vi "Data_get.vi"() -> ()   [LabVIEW 2009]
uses:
  <vilib>/Analysis/2dsp.llb/Real FFT.vi
  <vilib>/Analysis/NI_AALPro.lvlib
panel:
  in  "autoOFF":bool caption="Auto switch OFF"
  in  "SetRP":bool
  in  "Rep.Period":dbl=1.0 caption="Repetition Period(c)" min=1e-06 max=1000.0 step=0.1
  in  "PauseB":bool caption="Pause"
  in  "Substr":bool
  out "tdsavges#":i32 caption="tds averaged:"
  in  "Auto":bool caption="Autosave"
  in  "FFT every#":u32=1 min=1 max=1000 step=1
  in  "#steps":u32=1 min=1 step=1
  in  "f step (MHz)":dbl=0.0003 min=0.00025 max=67.0 step=1e-06 format="%#.12f"
  in  "ps/point":T1(ring)
  in  "ns/div":T2(ring)
  out "Current sweep":u32=1 min=1 max=1000 step=1
  in  "Ext":string="ccd"
  out "f cur. (MHz)":string
  in  "Name":string="trace"
  in  "Folder":path
  in  "#Sweeps":u32=1 min=1 max=1000 step=1
  in  "Ampl. (dBm)":dbl min=-135.0 max=30.0 step=0.5 format="%#_8g"
  in  "f start (MHz)":dbl=0.0003 min=0.00025 max=67.0 step=1e-06 format="%#.12f"
  in  "Start":bool
  in  "Quit":bool
  in  "E8257D VISA Port":refnum<visa-resource-name>="GPIB0::1::INSTR"
  out "read time (ms)":u32
  out "#points":u32
  out "Busy":bool
  in  "Repetition rate (Hz)":ext=2.5
  in  "Chirp start (MHz)":ext=2.5
  in  "Filter up to (MHz)":ext=2.5
  in  "Amount of averagings":u32=10 min=1 step=1
  out "Data":dbl[](array[numeric])
  out "XY Graph 5":cluster{ext[], dbl[]}(graph)
  out "FFT (Im)":dbl[](array[numeric])
  out "FFT (Re)":dbl[](array[numeric])
  out "Final array":ext[][](array[numeric])
  out "size(s)":i32
  out "Oscilloscope Data":dbl[](array[numeric])
  in  "Channel Number":u16=1
  out "Oscilloscope graph":dbl[](graph)
  in  "Stop":bool
  in  "TDS VISA Port":refnum<visa-resource-name>="GPIB0::1::INSTR"
  # "TDS6000"
  # "DG645"
  # "E8257D"
  # "File Storage"
  # "Control"
  # "Spectrum data"
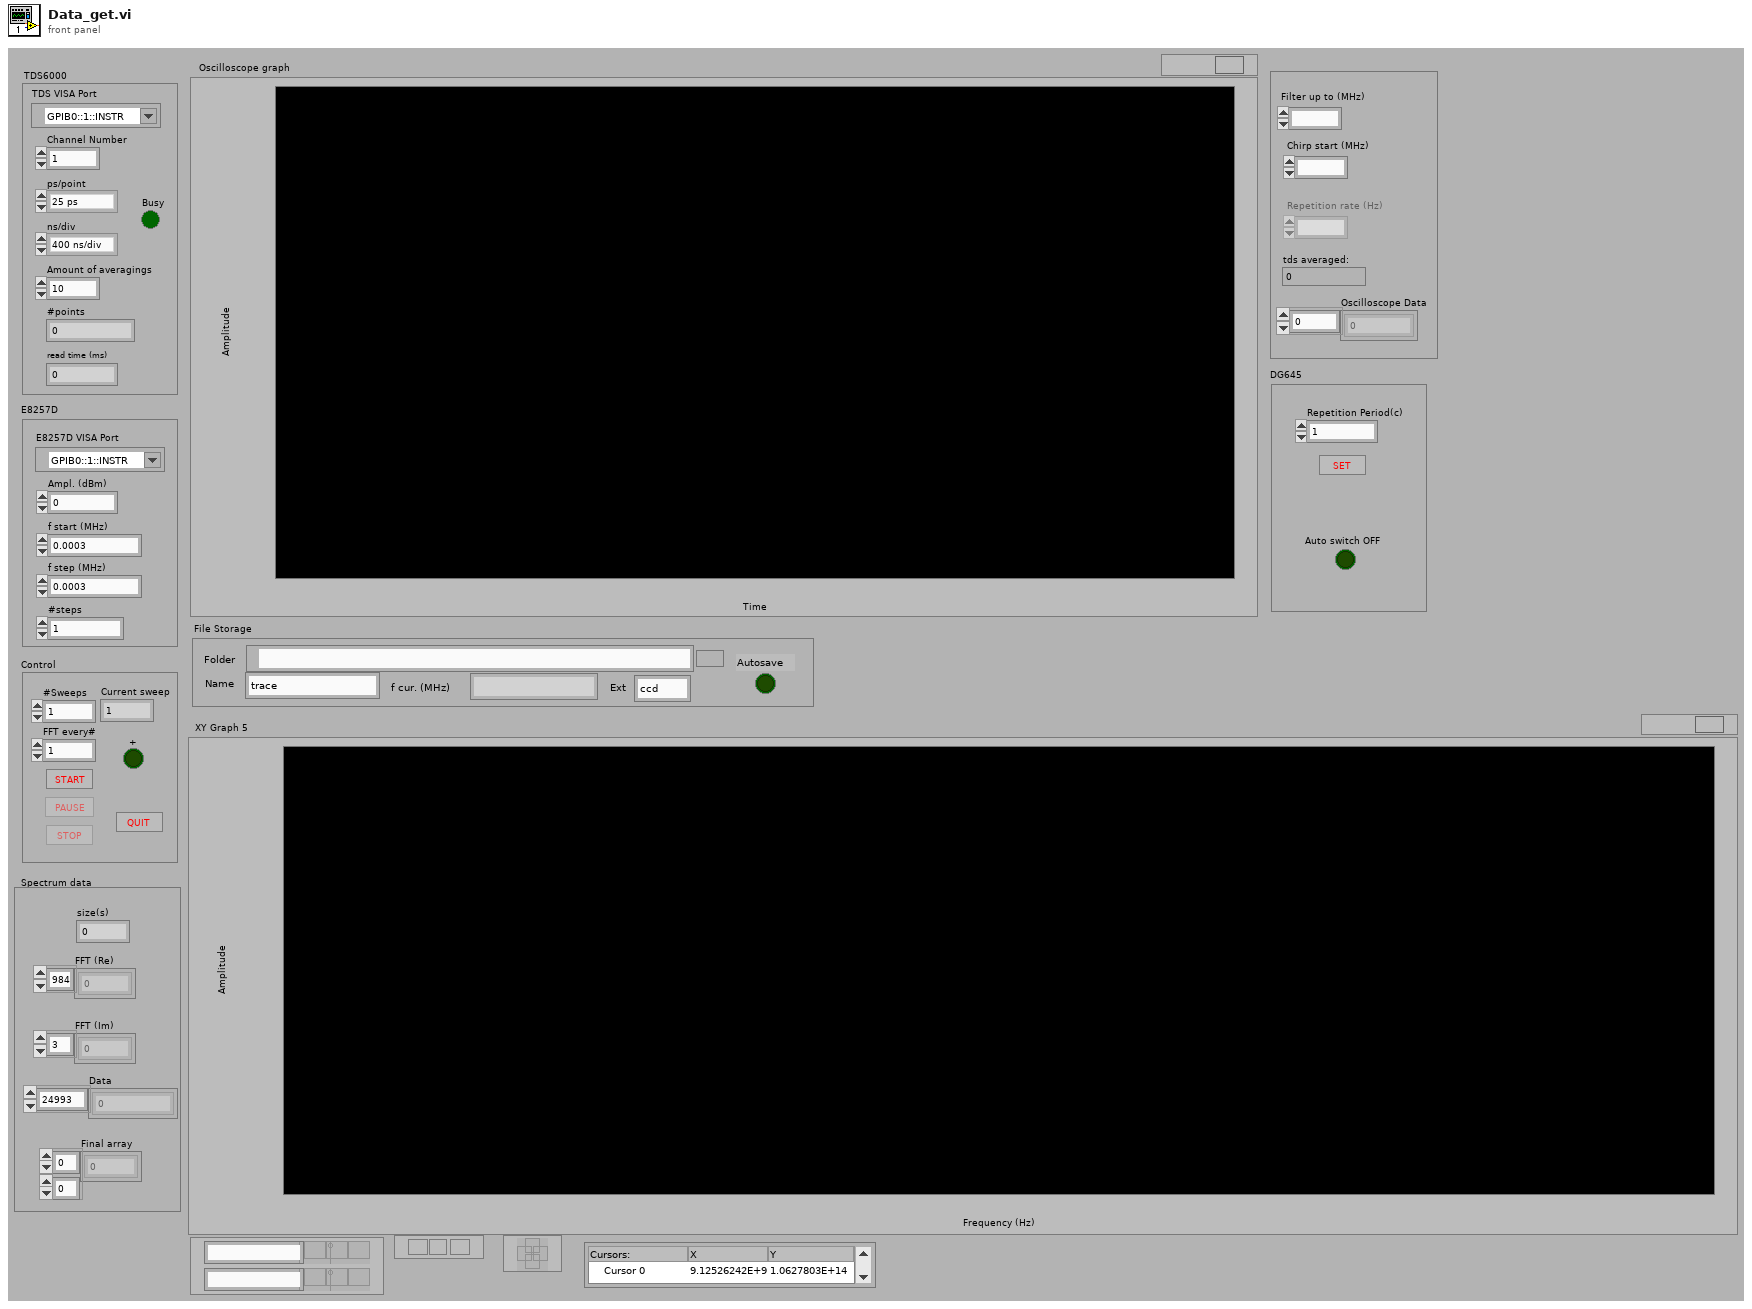
[diagram p1: front panel]
types:
  T1 = enum16{"25 ps", "50 ps", "100 ps", "200 ps", "400 ps", "800 ps", "2 ns"}
  T2 = enum16{"400 ns/div", "1 us/div", "2 us/div", "4 us/div", "10 us/div", "20 us/div"}
  T3 = enum8{"Enabled", "Disabled", "Disabled and Grayed Out"}
  T4 = enum16{"open", "replace", "create", "open or create", "replace or create", "replace or create with confirmation"}
  T5 = cluster{"Folder":path, "Name":string, "Ext":string}
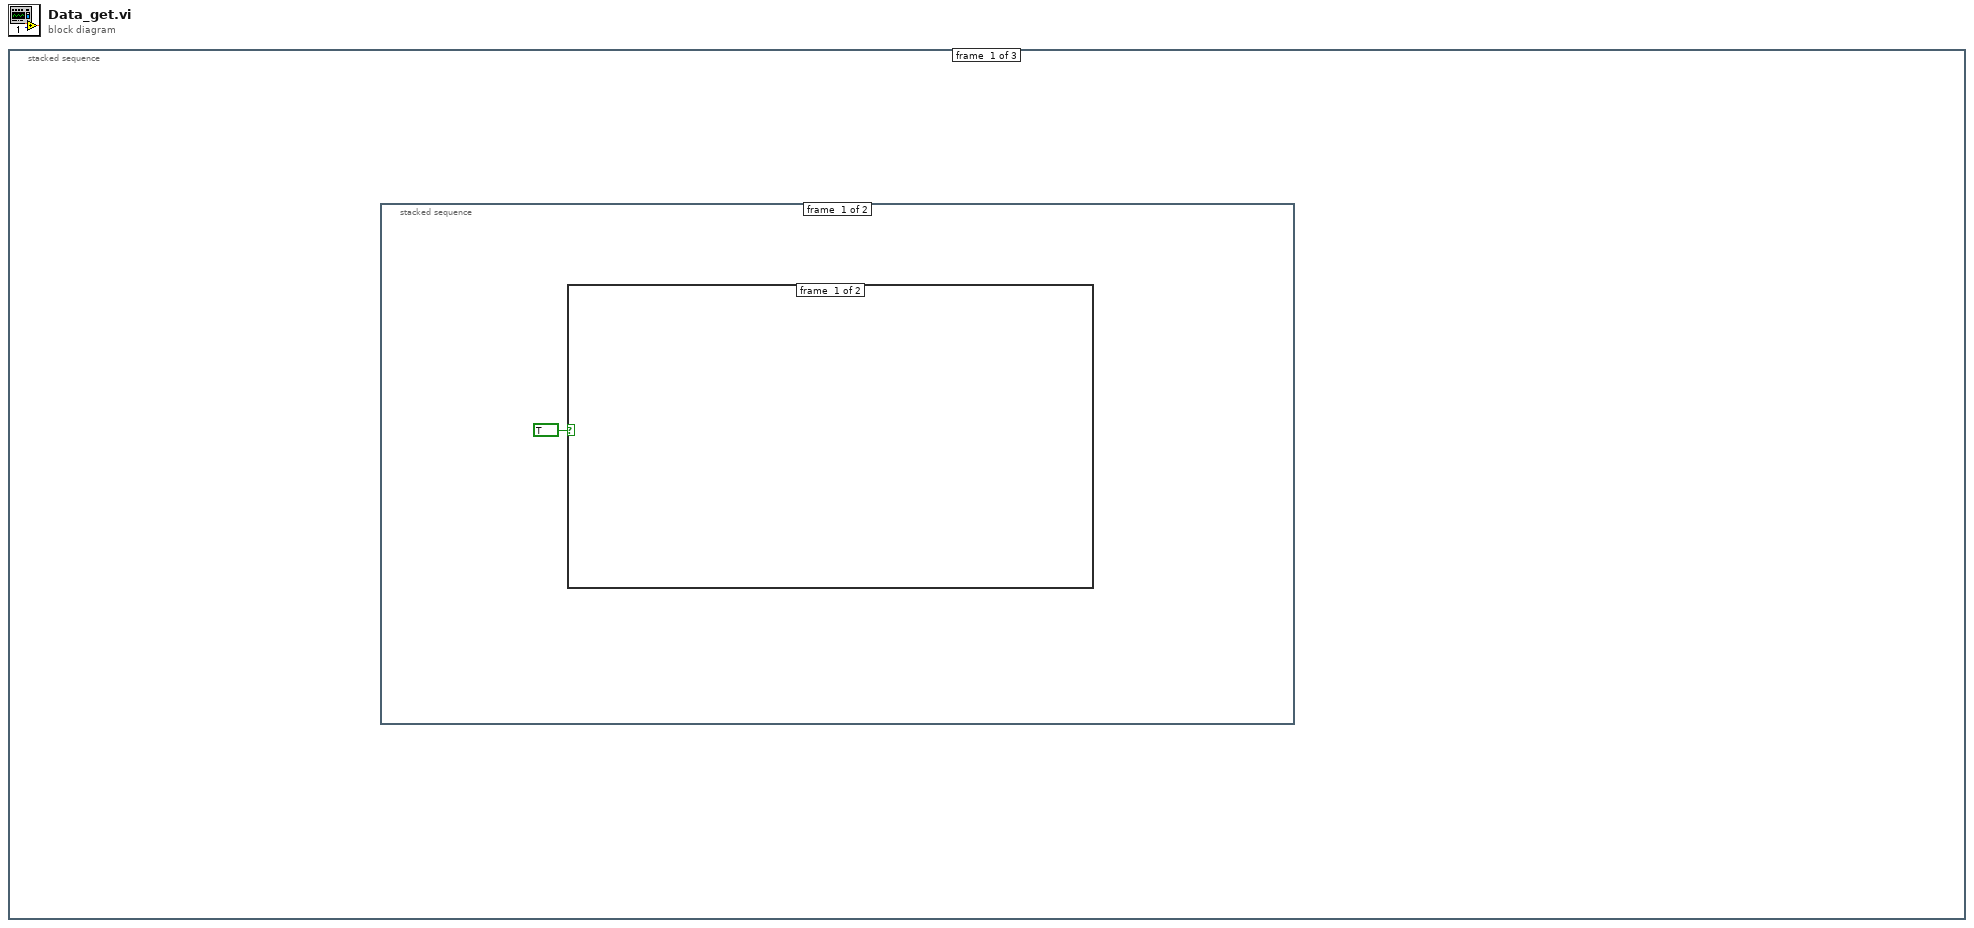
[diagram p0: block diagram]
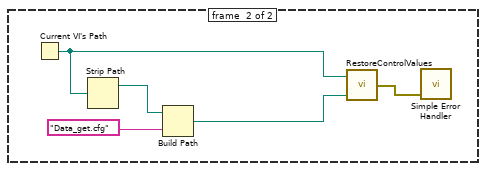
[diagram p2: hidden frame]
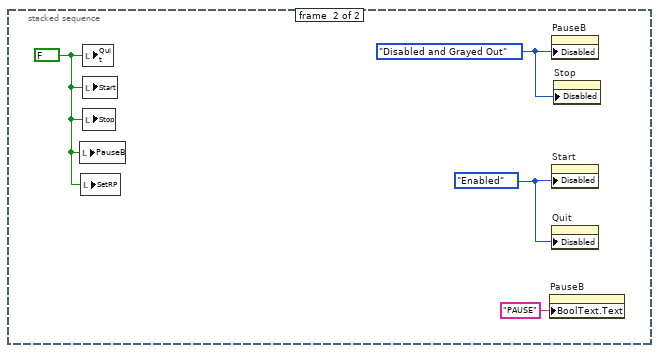
[diagram p3: hidden frame]
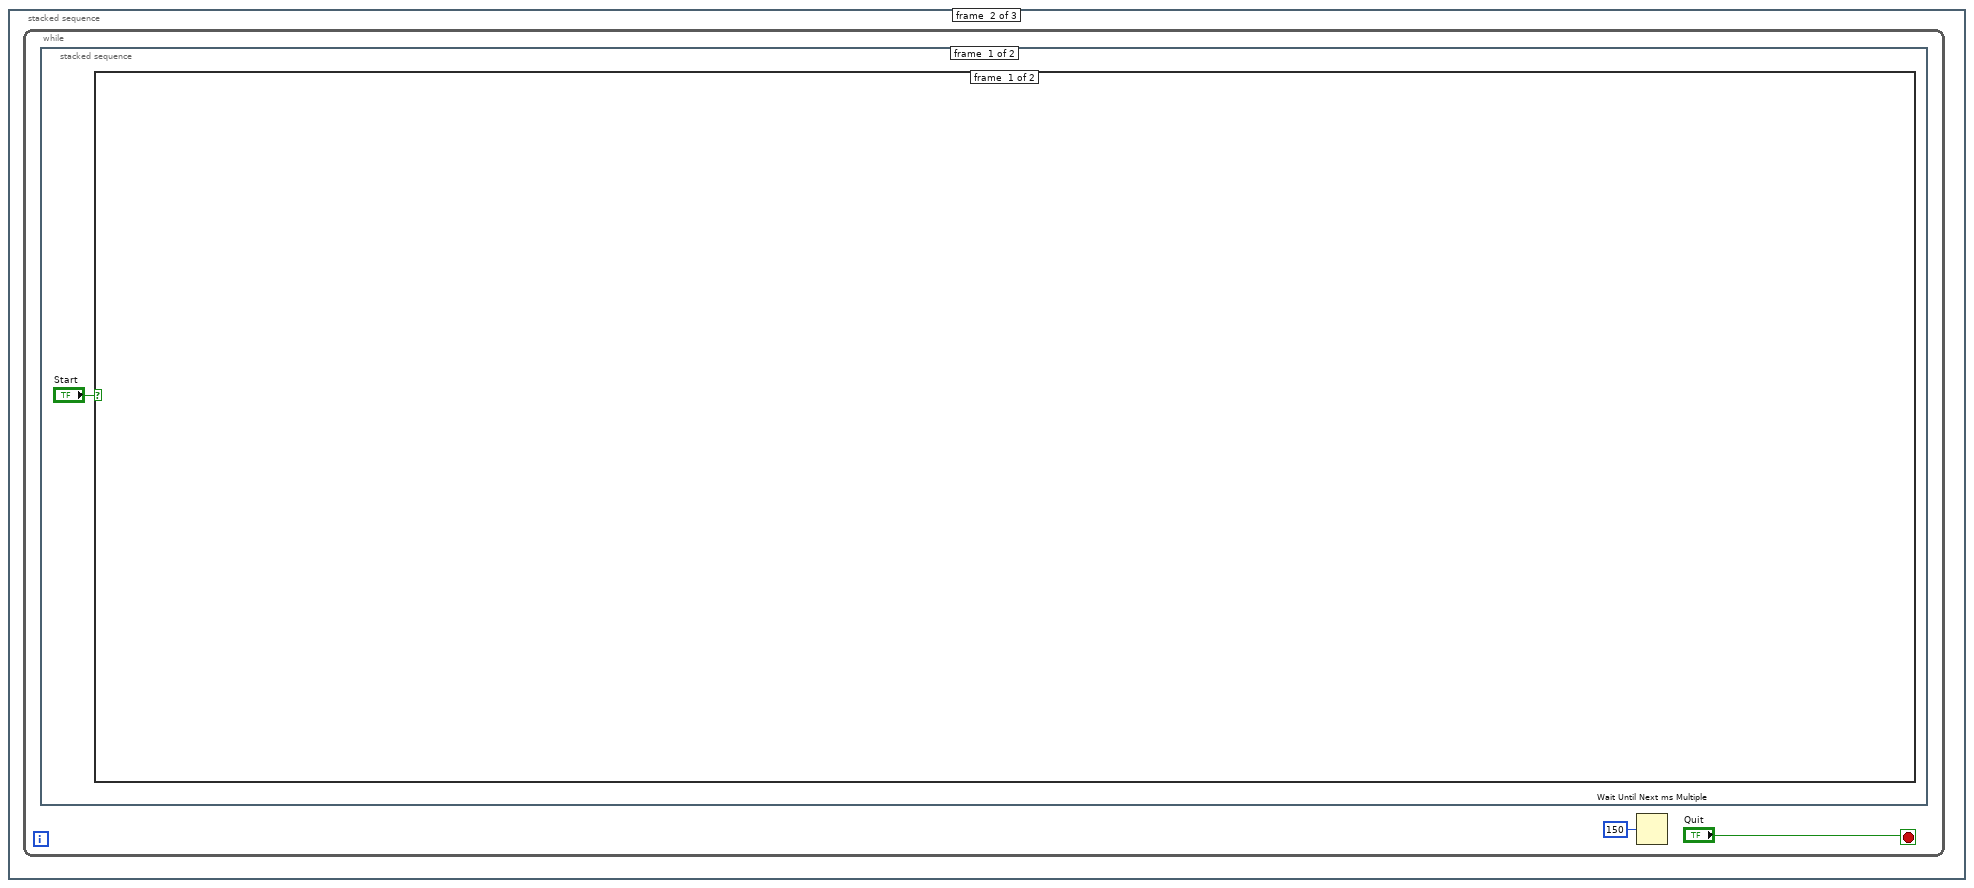
[diagram p4: hidden frame]
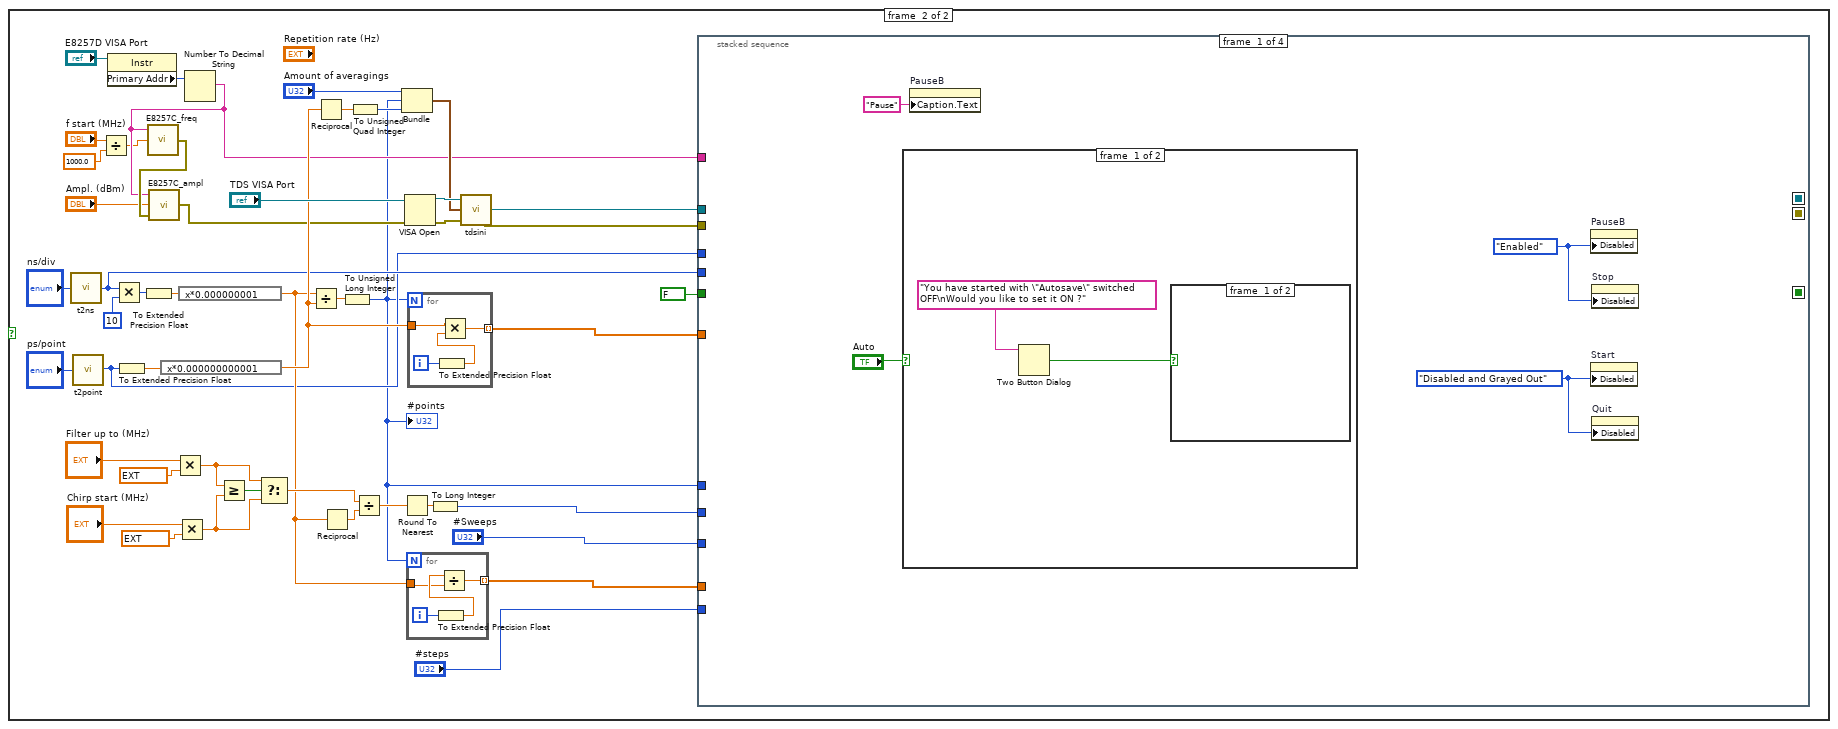
[diagram p5: hidden frame]
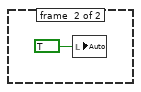
[diagram p6: hidden frame]
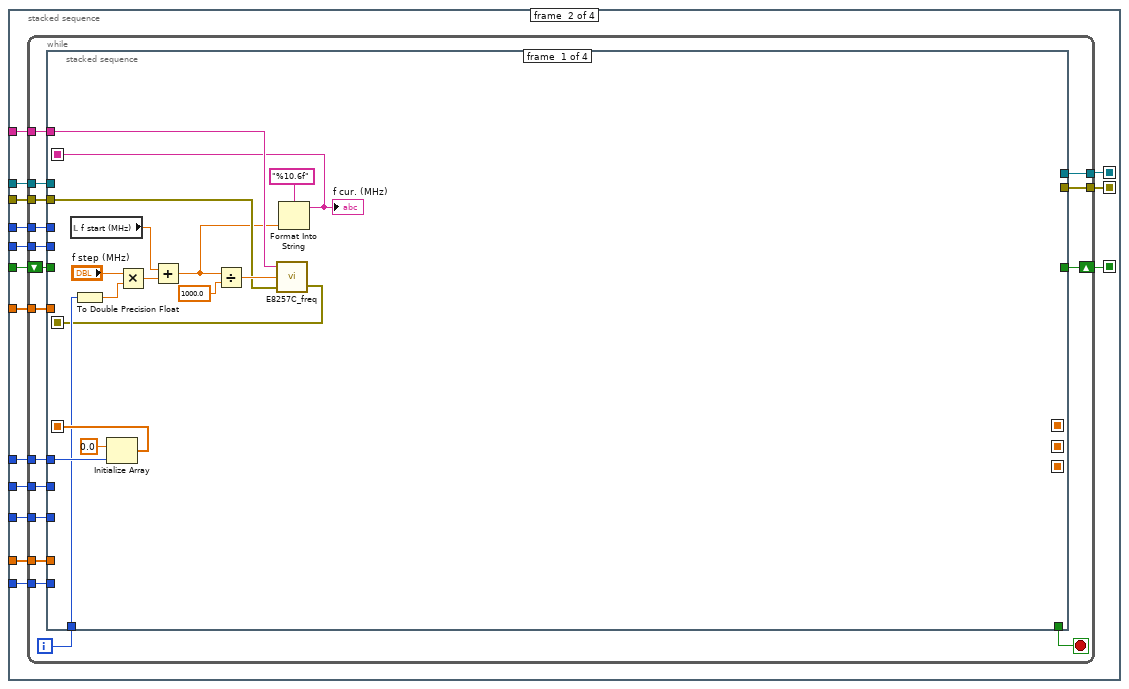
[diagram p8: hidden frame]
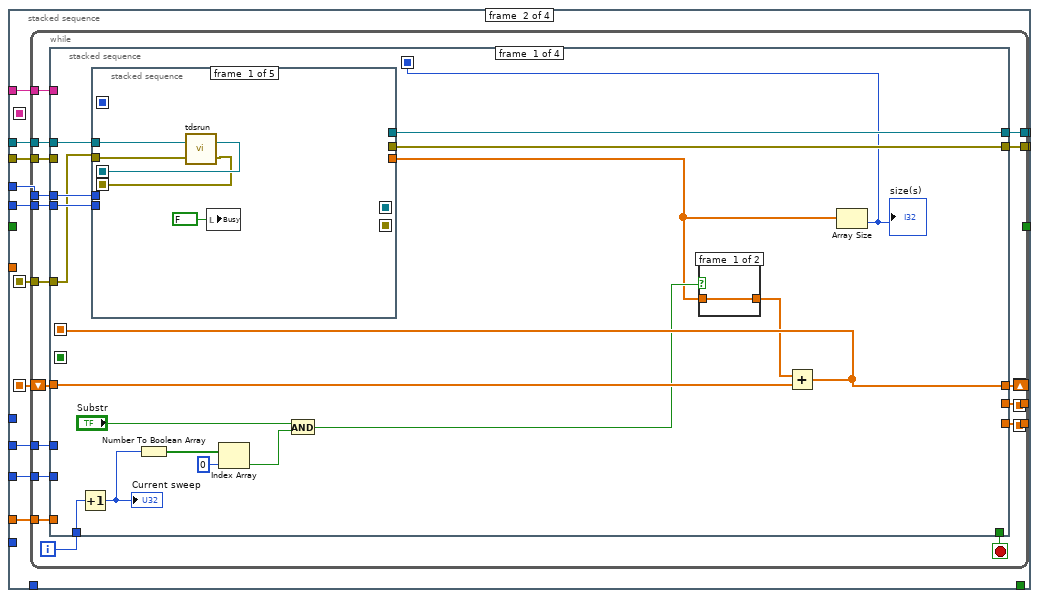
[diagram p9: hidden frame]
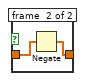
[diagram p10: hidden frame]
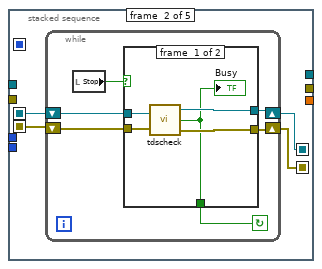
[diagram p11: hidden frame]
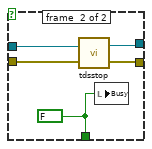
[diagram p12: hidden frame]
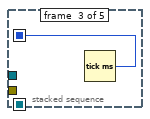
[diagram p13: hidden frame]
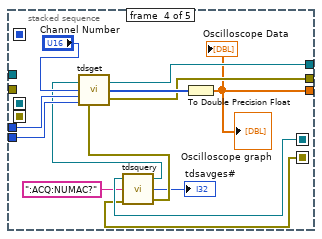
[diagram p14: hidden frame]
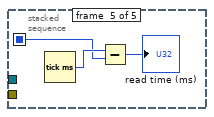
[diagram p15: hidden frame]
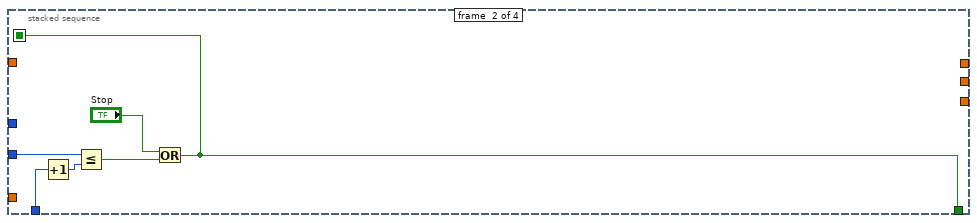
[diagram p16: hidden frame]
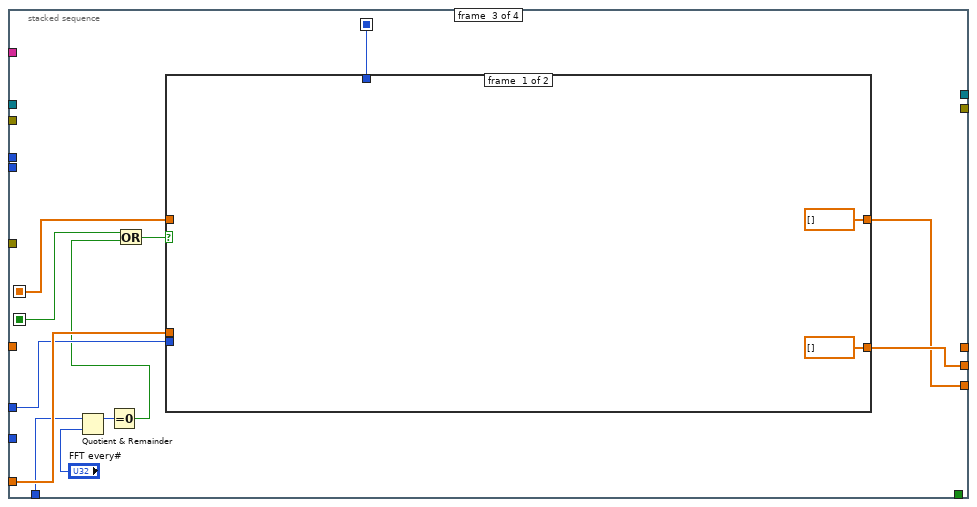
[diagram p17: hidden frame]
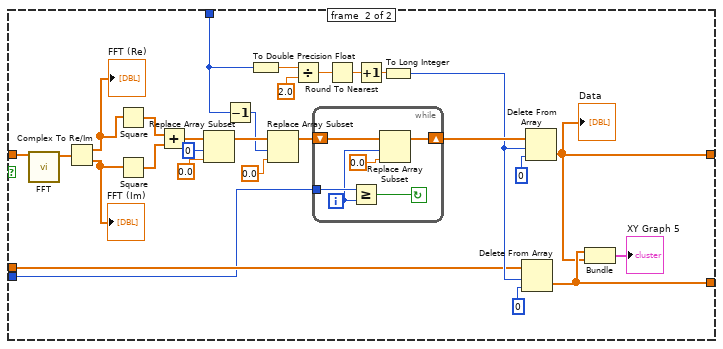
[diagram p18: hidden frame]
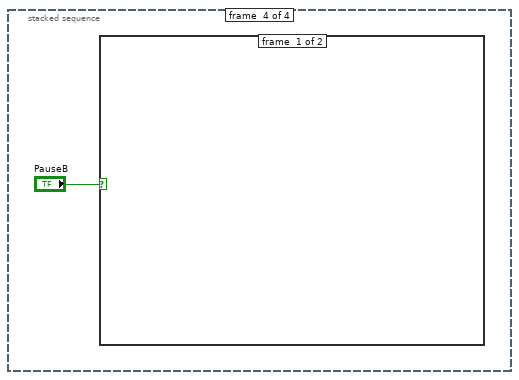
[diagram p19: hidden frame]
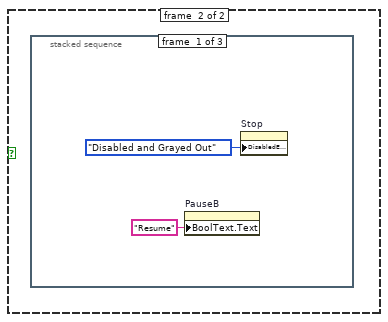
[diagram p20: hidden frame]
diagram:
  n1 = stacked-sequence {
    frame #0 {
      n2 = stacked-sequence {
        frame #0 {
          n3 = case shown="True" TRUE {
            frame #0 {
            }
            frame #1 {
              n4 = Current VI's Path() -> (path=w2:path)
              n5 = Strip Path(path=w2) -> (stripped path=w3:path)  [unwired: 1 out]
              n6 = Build Path(base path=w3, name or relative path="Data_get.cfg") -> (appended path=w5:path)
              n7 = call "RestoreControlValues.vi"("file path"=w5, "vi path"=w2) -> ("error out"=w4:errorcluster)
              n8 = call <vilib>:"Simple Error Handler.vi"("error in (no error)"=w4) -> ()  [unwired: 4 in, 5 out]
            }
          }
        }
        frame #1 {
          w10 = T3."Disabled and Grayed Out" ("Disabled")
          w8 = T3."Enabled" ("Disabled")
          w7 = FALSE ("Quit")
          n9 = local write "PauseB"(w7) -> ()
          n10 = local write "SetRP"(w7) -> ()
          n11 = local write "Quit"(w7) -> ()
          n12 = local write "Start"(w7) -> ()
          n13 = local write "Stop"(w7) -> ()
          n14 = property on="PauseB" class="Bool (strict)"("BoolText.Text"="PAUSE" ("Boolean Text.Text")) -> ()  [unwired: 2 in, 2 out]
          n15 = property on="PauseB" class="Bool (strict)"("Disabled"=w10) -> ()  [unwired: 2 in, 2 out]
          n16 = property on="Start" class="Bool (strict)"("Disabled"=w8) -> ()  [unwired: 2 in, 2 out]
          n17 = property on="Quit" class="Bool (strict)"("Disabled"=w8) -> ()  [unwired: 2 in, 2 out]
          n18 = property on="Stop" class="Bool (strict)"("Disabled"=w10) -> ()  [unwired: 2 in, 2 out]
        }
      }
    }
    frame #1 {
      n19 = while {
        stop <- "Quit" stop-if-true
        n20 = stacked-sequence {
          frame #0 {
            n21 = case shown="True" "Start" {
              frame #0 {
              }
              frame #1 {
                n22 = call "t2ns.vi"("t/div"="ns/div") -> ("ns/div"=w20:u32)
                n23 = call "t2point.vi"("t/point"="ps/point") -> ("ps/point"=w18:u32)
                n24 = Divide(x="f start (MHz)", y=1000.0) -> (x/y=w23:dbl)
                n25 = property class="Instr"(reference="E8257D VISA Port") -> ("Primary Addr"=w30:u16)  [unwired: 1 in, 2 out]
                n26 = Multiply(x=w20, y=u32 10) -> (x*y=w54:u32)
                n27 = To Extended Precision Float(1:w18) -> (0:w51:ext)
                n28 = To Extended Precision Float(1:w54) -> (0:w52:ext)
                n29 = expression code="x*0.000000000001"(w51) -> (w36:ext)
                n30 = Multiply(x="Filter up to (MHz)", y=ext 1000000.0) -> (x*y=w42:ext)
                n31 = Multiply(x="Chirp start (MHz)", y=ext 1000000.0) -> (x*y=w39:ext)
                n32 = expression code="x*0.000000001"(w52) -> (w32:ext)
                n33 = Number To Decimal String(number=w30) -> (decimal integer string=w27:string)  [unwired: 1 in]
                n34 = call "E8257C_freq.vi"("Frequency GHz"=w23, "GPIB address"=w27) -> ("error out"=w28:errorcluster)  [unwired: 1 in]
                n35 = call "E8257C_ampl.vi"("error in"=w28, "Amplitude dBm"="Ampl. (dBm)", "GPIB address"=w27) -> ("error out"=w26:errorcluster)
                n36 = Greater Or Equal?(x=w42, y=w39) -> (x >= y?=w50:bool)
                n37 = Select(t=w42, s=w50, f=w39) -> (s? t:f=w48:ext)
                n38 = Divide(x=w32, y=w36) -> (x/y=w53:ext)
                n39 = Reciprocal(x=w36) -> (1/x=w34:ext)
                n40 = Reciprocal(x=w32) -> (1/x=w49:ext)
                n41 = To Unsigned Long Integer(number=w53) -> (unsigned 32bit integer=w16:u32)
                "#points" <- w16
                n42 = To Unsigned Quad Integer(1:w34) -> (0:w35:u64)
                n43 = Divide(x=w48, y=w49) -> (x/y=w47:ext)
                n44 = Bundle("Amount of averagings"="Amount of averagings", w16, w35) -> (w37:cluster{"Amount of averagings ":u32, u32, u64})  [unwired: 1 in]
                n45 = Round To Nearest(number=w47) -> (nearest integer value=w46:ext)
                n46 = VISA Open(error in (no error)=w26, VISA resource name="TDS VISA Port") -> (VISA resource name=w57:refnum<visa-resource-name>, error out=w58:errorcluster)  [unwired: 3 in]
                n47 = for {
                  N: w16 -> [_]
                  tunnel: w32 -> [w455]
                  tunnel: [w457] -> w33 mode=indexing
                  i -> [w458]
                  n48 = To Extended Precision Float(1:w458) -> (0:w456:ext)
                  n49 = Divide(x=w456, y=w455) -> (x/y=w457:ext)
                }
                n50 = for {
                  N: w16 -> [_]
                  tunnel: w36 -> [w460]
                  tunnel: [w459] -> w21 mode=indexing
                  i -> [w462]
                  n51 = To Extended Precision Float(1:w462) -> (0:w461:ext)
                  n52 = Multiply(x=w460, y=w461) -> (x*y=w459:ext)
                }
                n53 = To Long Integer(number=w46) -> (32bit integer=w45:i32)
                n54 = call "tdsini.vi"("Error In (No Error)"=w58, "Acq_par"=w37, "VISA Port In"=w57) -> ("Error Out"=w59:errorcluster, "VISA Port Out"=w60:refnum<visa-resource-name>)
                n55 = stacked-sequence {
                  seq-local: [_ w74 _ _] -> [_ _ w410 _]
                  seq-local: [_ w73 _ _] -> [_ _ w409 _]
                  seq-local: [_ w68 _ _] -> [_ _ _ w417]
                  tunnel: w60 -> [_ w82 _ _]
                  tunnel: w59 -> [_ w81 _ _]
                  tunnel: w18 -> [_ w80 _ _]
                  tunnel: w20 -> [_ w79 _ _]
                  tunnel: w45 -> [_ w78 _ _]
                  tunnel: w33 -> [_ w77 _ _]
                  tunnel: w27 -> [_ w76 w407 _]
                  tunnel: "#Sweeps" -> [_ w75 _ _]
                  tunnel: w21 -> [_ w70 _ _]
                  tunnel: w16 -> [_ w72 _ _]
                  tunnel: "#steps" -> [_ w71 _ _]
                  tunnel: FALSE -> [_ w69 _ _]
                  frame #0 {
                    w62 = T3."Enabled" ("Disabled")
                    w61 = T3."Disabled and Grayed Out" ("Disabled")
                    n56 = case shown="False" "Auto" {
                      frame #0 {
                        n57 = Two Button Dialog(message="You have started with \"Autosave\" switched OFF\nWould you like to set it ON ?") -> (T button?=w65:bool)  [unwired: 2 in]
                        n58 = case shown="True" w65 {
                          frame #0 {
                          }
                          frame #1 {
                            n59 = local write "Auto"(TRUE) -> ()
                          }
                        }
                      }
                      frame #1 {
                      }
                    }
                    n60 = property on="PauseB" class="Bool (strict)"("Caption.Text"="Pause") -> ()  [unwired: 2 in, 2 out]
                    n61 = property on="PauseB" class="Bool (strict)"("Disabled"=w62) -> ()  [unwired: 2 in, 2 out]
                    n62 = property on="Start" class="Bool (strict)"("Disabled"=w61) -> ()  [unwired: 2 in, 2 out]
                    n63 = property on="Stop" class="Bool (strict)"("Disabled"=w62) -> ()  [unwired: 2 in, 2 out]
                    n64 = property on="Quit" class="Bool (strict)"("Disabled"=w61) -> ()  [unwired: 2 in, 2 out]
                  }
                  frame #1 {
                    n65 = while {
                      tunnel: w82 -> [w99]
                      tunnel: w81 -> [w98]
                      tunnel: w80 -> [w97]
                      tunnel: w79 -> [w96]
                      tunnel: w78 -> [w95]
                      tunnel: w77 -> [w94]
                      tunnel: w76 -> [w93]
                      tunnel: w75 -> [w92]
                      tunnel: [w91] -> w74
                      tunnel: [w90] -> w73
                      tunnel: w72 -> [w89]
                      tunnel: w71 -> [w87]
                      tunnel: w70 -> [w85]
                      shift-right: [w83] -> w68
                      shift-left: w69 -> [w84]
                      i -> [w88]
                      stop <- w86 stop-if-true
                      n66 = stacked-sequence {
                        seq-local: [w114 _ _ _] -> [_ w120 _ _]
                        seq-local: [w103 _ _ _] -> [_ w119 _ _]
                        seq-local: [_ w118 _ _] -> [_ _ w278 _]
                        seq-local: [_ w117 _ _] -> [_ _ w277 _]
                        seq-local: [_ w116 _ _] -> [_ _ w276 _]
                        seq-local: [w100 _ _ _] -> [_ _ w275 _]
                        tunnel: w99 -> [_ w130 _ _]
                        tunnel: w98 -> [w104 w129 _ _]
                        tunnel: w97 -> [_ w128 _ _]
                        tunnel: w96 -> [_ w127 _ _]
                        tunnel: w95 -> [_ w126 _ _]
                        tunnel: w94 -> [_ w125 _ _]
                        tunnel: w93 -> [w105 w124 _ _]
                        tunnel: w92 -> [_ w123 _ _]
                        tunnel: [_ w122 _ _] -> w91
                        tunnel: [_ w121 _ _] -> w90
                        tunnel: w89 -> [w113 _ _ _]
                        tunnel: w88 -> [w108 _ _ w400]
                        tunnel: w87 -> [_ _ _ w399]
                        tunnel: [_ _ _ w398] -> w86
                        tunnel: w85 -> [_ _ w279 _]
                        tunnel: w84 -> [_ _ w273 _]
                        tunnel: [_ _ w272 _] -> w83
                        frame #0 {
                          n67 = local read "f start (MHz)"() -> (w106:dbl)
                          n68 = To Double Precision Float(number=w108) -> (double precision float=w109:dbl)
                          n69 = Initialize Array(0.0 ("element"), w113) -> (w114:dbl[])
                          n70 = Multiply(x="f step (MHz)", y=w109) -> (x*y=w107:dbl)
                          n71 = Add(x=w106, y=w107) -> (x+y=w102:dbl)
                          n72 = Divide(x=w102, y=1000.0) -> (x/y=w112:dbl)
                          n73 = call "E8257C_freq.vi"("error in"=w104, "Frequency GHz"=w112, "GPIB address"=w105) -> ("error out"=w103:errorcluster)
                          n74 = Format Into String(format string="%10.6f", w102) -> (resulting string=w100:string)  [unwired: 2 in, 1 out]
                          "f cur. (MHz)" <- w100
                        }
                        frame #1 {
                          n75 = while {
                            tunnel: [w144] -> w121
                            tunnel: [w145] -> w122
                            tunnel: w129 -> [w146]
                            tunnel: w130 -> [w147]
                            tunnel: w128 -> [w143]
                            tunnel: w127 -> [w142]
                            tunnel: w125 -> [w140]
                            tunnel: w126 -> [w141]
                            tunnel: w124 -> [w137]
                            tunnel: w123 -> [w136]
                            shift-right: [w134] -> w118
                            shift-left: w120 -> [w135]
                            tunnel: [w133] -> w117
                            tunnel: w119 -> [w132]
                            tunnel: [w131] -> w116
                            i -> [w139]
                            stop <- w138 stop-if-true
                            n76 = stacked-sequence {
                              seq-local: [w157 _ _ _] -> [_ _ w228 _]
                              seq-local: [w158 _ _ _] -> [_ _ w227 _]
                              seq-local: [_ w211 _ _] -> [_ _ w218 _]
                              tunnel: w147 -> [w165 _ _ _]
                              tunnel: w146 -> [_ _ _ _]
                              tunnel: [w164 _ _ _] -> w145
                              tunnel: [w163 _ _ _] -> w144
                              tunnel: w143 -> [w162 _ _ _]
                              tunnel: w142 -> [w161 _ _ _]
                              tunnel: w141 -> [_ _ w225 _]
                              tunnel: w140 -> [_ _ w226 _]
                              tunnel: w139 -> [w156 w216 w222 _]
                              tunnel: [_ w211 _ _] -> w138
                              tunnel: w137 -> [_ _ _ _]
                              tunnel: w136 -> [_ w213 _ _]
                              tunnel: w135 -> [w160 _ _ _]
                              tunnel: [w158 _ _ _] -> w134
                              tunnel: [_ _ w224 _] -> w133
                              tunnel: w132 -> [w159 _ _ _]
                              tunnel: [_ _ w223 _] -> w131
                              frame #0 {
                                n77 = Increment(x=w156) -> (x+1=w148:i32)
                                "Current sweep" <- w148
                                n78 = stacked-sequence {
                                seq-local: [w171 _ _ _ _] -> [_ w177 _ _ _]
                                seq-local: [w170 _ _ _ _] -> [_ w176 _ _ _]
                                seq-local: [_ w174 _ _ _] -> [_ _ _ w199 _]
                                seq-local: [_ w175 _ _ _] -> [_ _ _ w200 _]
                                seq-local: [_ _ w194 _ _] -> [_ _ _ _ w209]
                                tunnel: w165 -> [w172 _ _ _ _]
                                tunnel: w159 -> [w173 _ _ _ _]
                                tunnel: [_ _ _ w206 _] -> w164
                                tunnel: [_ _ _ w205 _] -> w163
                                tunnel: w162 -> [_ _ _ w203 _]
                                tunnel: w161 -> [_ _ _ w202 _]
                                tunnel: [_ _ _ w201 _] -> w151
                                frame #0 {
                                n79 = call "tdsrun.vi"("Error In (No Error)"=w173, "VISA Port In"=w172) -> ("Error Out"=w170:errorcluster, "VISA Port Out"=w171:refnum<visa-resource-name>)
                                n80 = local write "Busy"(FALSE ("Busy")) -> ()
                                }
                                frame #1 {
                                n81 = while {
                                shift-right: [w181] -> w175
                                shift-left: w177 -> [w182]
                                shift-right: [w180] -> w174
                                shift-left: w176 -> [w183]
                                stop <- w179 continue-if-true
                                n82 = local read "Stop"() -> (w178:bool)
                                n83 = case shown="True" w178 {
                                tunnel: w183 -> [w188 w192]
                                tunnel: w182 -> [w187 w193]
                                tunnel: [w186 w190] -> w181
                                tunnel: [w185 w191] -> w180
                                tunnel: [w184 w189] -> w179
                                frame #0 {
                                n84 = call "tdscheck.vi"("VISA Port In"=w187, "Error In (No Error)"=w188) -> ("VISA Port Out"=w186:refnum<visa-resource-name>, "busy"=w184:bool, "Error Out"=w185:errorcluster)
                                "Busy" <- w184
                                }
                                frame #1 {
                                w189 = FALSE ("busy")
                                n85 = call "tdsstop.vi"("Error In (No Error)"=w192, "VISA Port In"=w193) -> ("Error Out"=w191:errorcluster, "VISA Port Out"=w190:refnum<visa-resource-name>)
                                n86 = local write "Busy"(w189) -> ()
                                }
                                }
                                }
                                }
                                frame #2 {
                                n87 = Tick Count (ms)() -> (millisecond timer value=w194:u32)
                                }
                                frame #3 {
                                n88 = call "tdsquery.vi"("Error In (No Error)"=w199, "String to TDS"=":ACQ:NUMAC?", "VISA Port In"=w200) -> ("Error Out"=w196:errorcluster, "number"=→"tdsavges#":i32, "VISA Port Out"=w197:refnum<visa-resource-name>)
                                n89 = call "tdsget.vi"("VISA Port In"=w197, "Channel Number"="Channel Number", "ps/point"=w203, "ns/div"=w202, "Error In (No Error)"=w196) -> ("VISA Port Out"=w206:refnum<visa-resource-name>, "TDS Data"=w207:u16[], "Error Out"=w205:errorcluster)  [unwired: 8 in]
                                n90 = To Double Precision Float(number=w207) -> (double precision float=w201:dbl[])
                                "Oscilloscope graph" <- w201
                                "Oscilloscope Data" <- w201
                                }
                                frame #4 {
                                n91 = Tick Count (ms)() -> (millisecond timer value=w210:u32)
                                n92 = Subtract(x=w210, y=w209) -> (x-y=→"read time (ms)":u32)
                                }
                                }
                                n93 = Number To Boolean Array(number=w148) -> (Boolean array=w155:bool[])
                                n94 = Index Array(array=w155, index=0) -> (element=w153:bool)
                                n95 = And(x="Substr", y=w153) -> (x .and. y?=w152:bool)
                                n96 = case shown="True" w152 {
                                tunnel: w151 -> [w166 w168]
                                tunnel: [w166 w167] -> w150
                                frame #0 {
                                }
                                frame #1 {
                                n97 = Negate(x=w168) -> (-x=w167:dbl[])
                                }
                                }
                                n98 = Add(x=w150, y=w160) -> (x+y=w158:dbl[])
                                n99 = Array Size(array=w151) -> (size(s)=w157:i32)
                                "size(s)" <- w157
                              }
                              frame #1 {
                                n100 = Increment(x=w216) -> (x+1=w212:i32)
                                n101 = Less Or Equal?(x=w213, y=w212) -> (x <= y?=w215:bool)
                                n102 = Or(x="Stop", y=w215) -> (x .or. y?=w211:bool)
                              }
                              frame #2 {
                                n103 = Quotient & Remainder(x=w222, y="FFT every#") -> (x-y*floor(x/y)=w220:u32)  [unwired: 1 out]
                                n104 = Equal To 0?(x=w220) -> (x = 0?=w217:bool)
                                n105 = Or(x=w218, y=w217) -> (x .or. y?=w219:bool)
                                n106 = case shown="True" w219 {
                                tunnel: w228 -> [_ w236]
                                tunnel: w227 -> [_ w235]
                                tunnel: w226 -> [_ w234]
                                tunnel: w225 -> [_ w233]
                                tunnel: [ext[] [] w232] -> w224
                                tunnel: [dbl[] [] w231] -> w223
                                frame #0 {
                                }
                                frame #1 {
                                n107 = call-poly <vilib>:"FFT.vi"("X"=w235) -> ("FFT {X}"=w258:cdb[])  [unwired: 9 in, 1 out]
                                n108 = Complex To Re/Im(x + iy=w258) -> (x=w257:dbl[], y=w256:dbl[])
                                "FFT (Re)" <- w257
                                "FFT (Im)" <- w256
                                n109 = Square(x=w257) -> (x^2=w255:dbl[])
                                n110 = Square(x=w256) -> (x^2=w254:dbl[])
                                n111 = Add(x=w255, y=w254) -> (x+y=w250:dbl[])
                                n112 = Replace Array Subset(array=w250, new element=0.0 ("new element/subarray"), index=0) -> (w249:dbl[])
                                n113 = Decrement(x=w236) -> (x-1=w248:i32)
                                n114 = To Double Precision Float(number=w236) -> (double precision float=w244:dbl)
                                n115 = Replace Array Subset(array=w249, new element=0.0 ("new element/subarray"), index=w248) -> (w246:dbl[])
                                n116 = Divide(x=w244, y=2.0) -> (x/y=w242:dbl)
                                n117 = while {
                                tunnel: w233 -> [w263]
                                shift-right: [w261] -> w245
                                shift-left: w246 -> [w262]
                                i -> [w260]
                                stop <- w264 continue-if-true
                                n118 = Greater Or Equal?(x=w263, y=w260) -> (x >= y?=w264:bool)
                                n119 = Replace Array Subset(array=w262, new element=0.0 ("new element/subarray"), index=w260) -> (w261:dbl[])
                                }
                                n120 = Round To Nearest(number=w242) -> (nearest integer value=w241:dbl)
                                n121 = Increment(x=w241) -> (x+1=w240:dbl)
                                n122 = To Long Integer(number=w240) -> (32bit integer=w237:i32)
                                n123 = Delete From Array(array=w234, length=w237, index=0) -> (deleted portion=w232:ext[])  [unwired: 1 out]
                                n124 = Delete From Array(array=w245, length=w237, index=0) -> (deleted portion=w231:dbl[])  [unwired: 1 out]
                                "Data" <- w231
                                n125 = Bundle(w232, w231) -> (→"XY Graph 5":cluster{ext[], dbl[]})  [unwired: 1 in]
                                }
                                }
                              }
                              frame #3 {
                                n126 = case shown="True" "PauseB" {
                                frame #0 {
                                }
                                frame #1 {
                                n127 = stacked-sequence {
                                frame #0 {
                                n128 = property on="PauseB" class="Bool (strict)"("BoolText.Text"="Resume" ("Caption.Text")) -> ()  [unwired: 2 in, 2 out]
                                n129 = property on="Stop" class="Bool (strict)"("DisabledEnum"=T3."Disabled and Grayed Out" ("Disabled")) -> ()  [unwired: 2 in, 2 out]
                                }
                                frame #1 {
                                n130 = while {
                                stop <- w269 continue-if-true
                                n131 = local read "PauseB"() -> (w269:bool)
                                n132 = Wait Until Next ms Multiple(millisecond multiple=u32 150) -> ()  [unwired: 1 out]
                                }
                                }
                                frame #2 {
                                n133 = property on="PauseB" class="Bool (strict)"("BoolText.Text"="Pause" ("Caption.Text")) -> ()  [unwired: 2 in, 2 out]
                                n134 = property on="Stop" class="Bool (strict)"("DisabledEnum"=T3."Enabled" ("Disabled")) -> ()  [unwired: 2 in, 2 out]
                                }
                                }
                                }
                                }
                              }
                            }
                          }
                        }
                        frame #2 {
                          n135 = local read "Auto"() -> (w274:bool)
                          n136 = case shown="True" w274 {
                            tunnel: w279 -> [_ w287]
                            tunnel: w278 -> [_ w286]
                            tunnel: w277 -> [_ w285]
                            tunnel: w276 -> [_ w284]
                            tunnel: w275 -> [_ w283]
                            tunnel: w273 -> [_ w282]
                            tunnel: [FALSE w281] -> w272
                            frame #0 {
                            }
                            frame #1 {
                              n137 = stacked-sequence {
                                seq-local: [w288 _ _ _] -> [_ w313 _ _]
                                seq-local: [_ _ w368 _] -> [_ _ _ w389]
                                seq-local: [_ w300 _ _] -> [_ _ _ w380]
                                tunnel: w287 -> [_ w315 _ _]
                                tunnel: w286 -> [_ w302 _ _]
                                tunnel: w285 -> [_ _ _ w392]
                                tunnel: w284 -> [_ _ _ w391]
                                tunnel: w283 -> [w290 w301 w370 _]
                                tunnel: w282 -> [_ w305 _ _]
                                tunnel: [_ w300 _ _] -> w281
                                frame #0 {
                                n138 = Path To String(path="Folder") -> (string=w298:string)
                                n139 = Concatenate Strings(w298, "\\\\" ("string"), "Name", "_") -> (w289:string)
                                n140 = Concatenate Strings(w289, "td", w290, ".", "Ext") -> (w288:string)
                                }
                                frame #1 {
                                n141 = String To Path(string=w313) -> (path=w304:path)
                                n142 = case shown="False" w305 {
                                tunnel: w313 -> [w319 _]
                                tunnel: [w324 w366] -> w300
                                tunnel: [w322 T4."replace or create" ("operation (0:open)")] -> w307
                                tunnel: w305 -> [w323 w366]
                                tunnel: w304 -> [w321 w365]
                                tunnel: [w320 w365] -> w303
                                tunnel: w301 -> [w318 _]
                                frame #0 {
                                n143 = call "CheckFileExist.vi"("Path"=w319) -> ("Exist"=w326:bool, "Overwrite"=w325:bool)  [unwired: 1 in, 1 out]
                                n144 = case shown="True" w326 {
                                tunnel: w325 -> [_ w335]
                                tunnel: [w329 w333] -> w324
                                tunnel: w323 -> [w329 _]
                                tunnel: [T4."create" ("operation (0:open)") w334] -> w322
                                tunnel: w321 -> [w327 w332]
                                tunnel: [w327 w331] -> w320
                                tunnel: w318 -> [_ w330]
                                frame #0 {
                                }
                                frame #1 {
                                n145 = case shown="True" w335 {
                                tunnel: [w338 T4."replace or create" ("operation (0:open)")] -> w334
                                tunnel: [w339 TRUE] -> w333
                                tunnel: w332 -> [_ w362]
                                tunnel: [w336 w362] -> w331
                                tunnel: w330 -> [w337 _]
                                frame #0 {
                                n146 = stacked-sequence {
                                tunnel: [_ _ FALSE] -> w339
                                tunnel: [_ _ T4."create" ("operation (0:open)")] -> w338
                                tunnel: w337 -> [_ w351 _]
                                tunnel: [_ w348 _] -> w336
                                frame #0 {
                                n147 = local read "Folder"() -> (w347:path)
                                n148 = local read "Name"() -> (w346:string)
                                n149 = local read "Ext"() -> (w345:string)
                                n150 = Bundle("Folder"=w347, "Name"=w346, "Ext"=w345) -> (w344:T5)  [unwired: 1 in]
                                n151 = call "ChangeFileName.vi"("input par"=w344) -> ("output par"=w343:T5)  [unwired: 1 out]
                                n152 = Unbundle(w343) -> ("Folder"=w342:path, "Name"=w341:string, "Ext"=w340:string)
                                n153 = local write "Folder"(w342) -> ()
                                n154 = local write "Name"(w341) -> ()
                                n155 = local write "Ext"(w340) -> ()
                                }
                                frame #1 {
                                n156 = local read "Folder"() -> (w356:path)
                                n157 = local read "Name"() -> (w355:string)
                                n158 = local read "Ext"() -> (w350:string)
                                n159 = Path To String(path=w356) -> (string=w359:string)
                                n160 = Concatenate Strings(w359, "\\\\" ("string"), w355, "_") -> (w352:string)
                                n161 = Concatenate Strings(w352, "td", w351, ".", w350) -> (w349:string)
                                n162 = String To Path(string=w349) -> (path=w348:path)
                                }
                                frame #2 {
                                }
                                }
                                }
                                frame #1 {
                                }
                                }
                                }
                                }
                                }
                                frame #1 {
                                }
                                }
                                n163 = Build Array(w315, w302) -> (w317:ext[][])
                                n164 = Transpose 2D Array(2D array=w317) -> (transposed array=w314:ext[][])
                                n165 = Array To Spreadsheet String(array=w314, 3:"%e") -> (spreadsheet string=w306:string)  [unwired: 1 in]
                                n166 = Open/Create/Replace File(file path (use dialog)=w303, operation (0:open)=w307, access (0:read/write)=enum16{"read/write", "read-only", "write-only"}."write-only") -> (refnum out=w309:refnum<file>, error out=w312:errorcluster)  [unwired: 3 in, 1 out]
                                n167 = Write to Text File(file (use dialog)=w309, text=w306, error in=w312) -> (refnum out=w310:refnum<file>, error out=w311:errorcluster)  [unwired: 1 in, 1 out]
                                n168 = Close File(refnum=w310, error in=w311) -> (error out=w299:errorcluster)  [unwired: 1 out]
                                n169 = call <vilib>:"Simple Error Handler.vi"("error in (no error)"=w299) -> ()  [unwired: 4 in, 5 out]
                                }
                                frame #2 {
                                n170 = local read "Folder"() -> (w372:path)
                                n171 = local read "Name"() -> (w371:string)
                                n172 = local read "Ext"() -> (w369:string)
                                n173 = Path To String(path=w372) -> (string=w378:string)
                                n174 = Concatenate Strings(w378, "\\\\" ("string"), w371, "_") -> (w373:string)
                                n175 = Concatenate Strings(w373, "sd", w370, ".", w369) -> (w368:string)
                                }
                                frame #3 {
                                n176 = To Extended Precision Float(1:w391) -> (0:w393:ext[])
                                n177 = String To Path(string=w389) -> (path=w382:path)
                                n178 = case shown="True" w380 {
                                tunnel: [T4."replace or create with confirmation" ("operation (0:open)") T4."replace or create" ("operation (0:open)")] -> w381
                                frame #0 {
                                }
                                frame #1 {
                                }
                                }
                                n179 = Build Array(w392, w393) -> (w390:ext[][])
                                n180 = Transpose 2D Array(2D array=w390) -> (transposed array=w394:ext[][])
                                "Final array" <- w394
                                n181 = Array To Spreadsheet String(array=w394, 3:"%e") -> (spreadsheet string=w383:string)  [unwired: 1 in]
                                n182 = Open/Create/Replace File(file path (use dialog)=w382, operation (0:open)=w381, access (0:read/write)=enum16{"read/write", "read-only", "write-only"}."write-only") -> (refnum out=w385:refnum<file>, error out=w388:errorcluster)  [unwired: 3 in, 1 out]
                                n183 = Write to Text File(file (use dialog)=w385, text=w383, error in=w388) -> (refnum out=w386:refnum<file>, error out=w387:errorcluster)  [unwired: 1 in, 1 out]
                                n184 = Close File(refnum=w386, error in=w387) -> (error out=w379:errorcluster)  [unwired: 1 out]
                                n185 = call <vilib>:"Simple Error Handler.vi"("error in (no error)"=w379) -> ()  [unwired: 4 in, 5 out]
                                }
                              }
                            }
                          }
                        }
                        frame #3 {
                          n186 = Increment(x=w400) -> (x+1=w402:i32)
                          n187 = Less Or Equal?(x=w399, y=w402) -> (x <= y?=w403:bool)
                          n188 = local read "Stop"() -> (w401:bool)
                          n189 = Or(x=w401, y=w403) -> (x .or. y?=w398:bool)
                        }
                      }
                    }
                  }
                  frame #2 {
                    w406 = T3."Disabled and Grayed Out" ("Disabled")
                    w405 = T3."Enabled" ("Disabled")
                    n190 = call "E8257C_local.vi"("GPIB address"=w407) -> ("error out"=w408:errorcluster)  [unwired: 1 in]
                    n191 = call <vilib>:"Simple Error Handler.vi"("error in (no error)"=w408) -> ()  [unwired: 4 in, 5 out]
                    n192 = property on="Quit" class="Bool (strict)"("Disabled"=w405) -> ()  [unwired: 2 in, 2 out]
                    n193 = property on="PauseB" class="Bool (strict)"("Disabled"=w406) -> ()  [unwired: 2 in, 2 out]
                    n194 = property on="Stop" class="Bool (strict)"("Disabled"=w406) -> ()  [unwired: 2 in, 2 out]
                    n195 = property on="Start" class="Bool (strict)"("Disabled"=w405) -> ()  [unwired: 2 in, 2 out]
                    n196 = case shown="True" "autoOFF" {
                      frame #0 {
                      }
                      frame #1 {
                        w415 = u32 1 items=["internal", "external", "single shot", "burst", "line"] ("trigger")
                        n197 = call "dg535 trigger.vi"("external trigger level"=sgl 10.0, "trigger slope"=FALSE, "input impedance"=FALSE, "trigger"=w415, "GPIB address"="15") -> ("error out"=w412:errorcluster)  [unwired: 4 in]
                        n198 = call <vilib>:"Simple Error Handler.vi"("error in (no error)"=w412) -> ()  [unwired: 4 in, 5 out]
                      }
                    }
                    n199 = VISA Close(VISA resource name=w410, error in (no error)=w409) -> ()  [unwired: 1 out]
                  }
                  frame #3 {
                    n200 = local read "Auto"() -> (w418:bool)
                    n201 = case shown="True" w418 {
                      tunnel: w417 -> [_ w421]
                      frame #0 {
                      }
                      frame #1 {
                        n202 = local read "Channel Number"() -> (w451:u16)
                        n203 = local read "ps/point"() -> (w450:T1)
                        n204 = local read "ns/div"() -> (w449:T2)
                        n205 = local read "Amount of averagings"() -> (w448:u32)
                        n206 = local read "#Sweeps"() -> (w447:u32)
                        n207 = local read "Filter up to (MHz)"() -> (w446:ext)
                        n208 = local read "Chirp start (MHz)"() -> (w445:ext)
                        n209 = local read "Ampl. (dBm)"() -> (w444:dbl)
                        n210 = local read "f start (MHz)"() -> (w441:dbl)
                        n211 = local read "f step (MHz)"() -> (w440:dbl)
                        n212 = local read "#steps"() -> (w439:u32)
                        n213 = call "t2point.vi"("t/point"=w450) -> ("ps/point"=w442:u32)
                        n214 = call "t2ns.vi"("t/div"=w449) -> ("ns/div"=w443:u32)
                        n215 = local read "Folder"() -> (w435:path)
                        n216 = local read "Name"() -> (w434:string)
                        n217 = local read "Ext"() -> (w431:string)
                        n218 = Path To String(path=w435) -> (string=w438:string)
                        n219 = Format Into String(format string="Channel: %d\\nps/point: %d\\nns/div: %d\\nAmount of averagings: %d\\n#Sweeps: %d\\nFilter up to (MHz): %f\\nChirp start (MHz): %f\\nAmpl. (dBm): %f\\nf start (MHz): %f\\nf step (MHz): %f\\n#steps: %d\\n", w451, w442, w443, w448, w447, w446, w445, w444, w441, w440, w439) -> (resulting string=w422:string)  [unwired: 2 in, 1 out]
                        n220 = Concatenate Strings(w438, "\\\\" ("string"), w434, "_", "par", ".", w431) -> (w430:string)
                        n221 = case shown="False" w421 {
                          tunnel: [T4."replace or create with confirmation" ("operation (0:open)") T4."replace or create" ("operation (0:open)")] -> w420
                          frame #0 {
                          }
                          frame #1 {
                          }
                        }
                        n222 = String To Path(string=w430) -> (path=w424:path)
                        n223 = Open/Create/Replace File(file path (use dialog)=w424, operation (0:open)=w420, access (0:read/write)=enum16{"read/write", "read-only", "write-only"}."write-only") -> (refnum out=w426:refnum<file>, error out=w429:errorcluster)  [unwired: 3 in, 1 out]
                        n224 = Write to Text File(file (use dialog)=w426, text=w422, error in=w429) -> (refnum out=w427:refnum<file>, error out=w428:errorcluster)  [unwired: 1 in, 1 out]
                        n225 = Close File(refnum=w427, error in=w428) -> (error out=w425:errorcluster)  [unwired: 1 out]
                        n226 = call <vilib>:"Simple Error Handler.vi"("error in (no error)"=w425) -> ()  [unwired: 4 in, 5 out]
                      }
                    }
                    n227 = local write "Stop"(FALSE ("Stop")) -> ()
                  }
                }
              }
            }
          }
          frame #1 {
            n228 = case shown="True" "SetRP" {
              frame #0 {
              }
              frame #1 {
                n229 = stacked-sequence {
                  frame #0 {
                    w466 = u32 0 items=["internal", "external", "single shot", "burst", "line"] ("trigger")
                    n230 = Reciprocal(x="Rep.Period") -> (1/x=w465:dbl)
                    n231 = call "dg535 trigger.vi"("internal/burst trigger rate"=w465, "trigger"=w466, "GPIB address"="15") -> ("error out"=w464:errorcluster)  [unwired: 6 in]
                    n232 = call <vilib>:"Simple Error Handler.vi"("error in (no error)"=w464) -> ()  [unwired: 4 in, 5 out]
                  }
                  frame #1 {
                    n233 = local write "SetRP"(FALSE ("SetRP")) -> ()
                  }
                }
              }
            }
          }
        }
        n234 = Wait Until Next ms Multiple(millisecond multiple=u32 150) -> ()  [unwired: 1 out]
      }
    }
    frame #2 {
      n235 = Current VI's Path() -> (path=w470:path)
      n236 = Strip Path(path=w470) -> (stripped path=w471:path)  [unwired: 1 out]
      n237 = Build Path(base path=w471, name or relative path="Data_get.cfg") -> (appended path=w473:path)
      n238 = call "SaveControlValues.vi"("file path"=w473, "vi path"=w470) -> ("error out"=w472:errorcluster)
      n239 = call <vilib>:"Simple Error Handler.vi"("error in (no error)"=w472) -> ()  [unwired: 4 in, 5 out]
    }
  }
